vi "Check Filter Repositioning Status.vi"(0 "Session Handle in":T1, 11 "error in (no error)":errorcluster) -> (4 "Session Handle out":T1, 6 "Success?":bool, 15 "error out":errorcluster)   [LabVIEW 2015, in "PAS.lvclass"]
uses:
  PAS.lvclass
  Typedefs/Session Handle.ctl
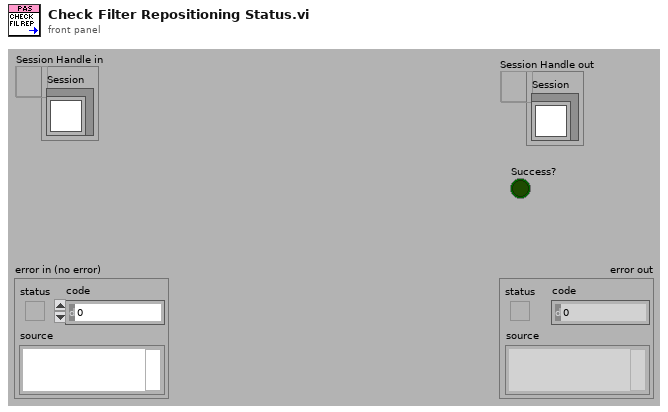
[diagram p1: front panel]
types:
  T1 = typedef "PAS.lvclass/Session Handle.ctl" = refnum<data-value>
  T2 = typedef "XNET Frame CAN.ctl" = cluster{"timestamp":timestamp, "payload":u8[], "identifier":u32, "type":T3, "extended?":bool, "echo?":bool}
  T3 = typedef "XNET Frame Type CAN.ctl" = u8
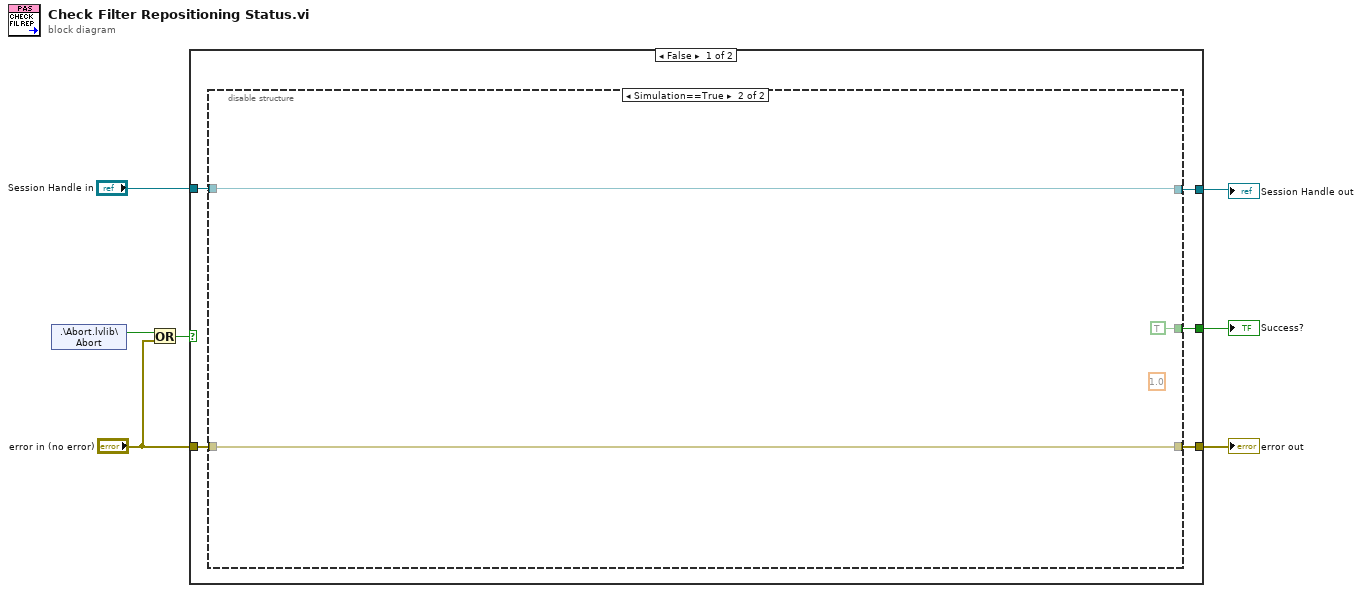
[diagram p0: block diagram]
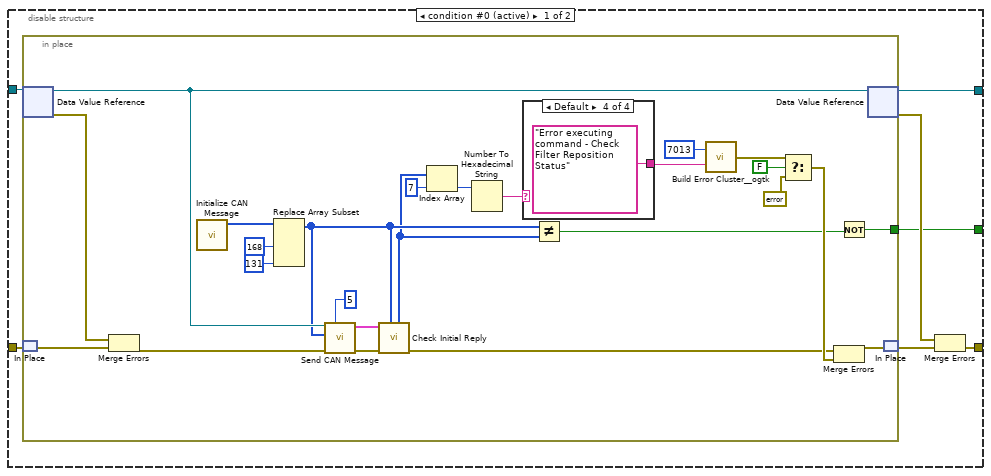
[diagram p2: hidden frame]
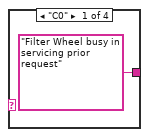
[diagram p3: hidden frame]
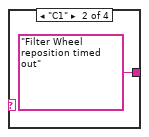
[diagram p4: hidden frame]
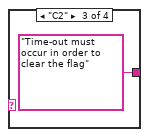
[diagram p5: hidden frame]
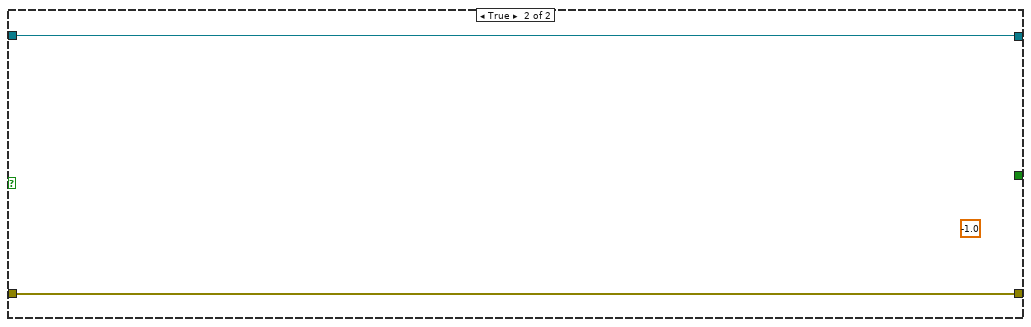
[diagram p6: hidden frame]
diagram:
  n1 = shared-variable ".\\Abort.lvlib\\Abort"() -> (w4:bool)  [unwired: 1 in, 1 out]
  n2 = Or(x=w4, y="error in (no error)") -> (x .or. y?=w2:bool)
  n3 = case shown="False" w2 {
    tunnel: [w12 w53] -> w6
    tunnel: [w11 w52] -> w5
    tunnel: "Session Handle in" -> [w10 w53]
    tunnel: "error in (no error)" -> [w9 w52]
    tunnel: [w8 _] -> w1
    frame False {
      n4 = disable-structure shown="Simulation==True" {
        disable-tunnel: [w19 w51] -> w12
        disable-tunnel: [w16 w50] -> w11
        disable-tunnel: w10 -> [w15 w51]
        disable-tunnel: w9 -> [w14 w50]
        disable-tunnel: [w13 TRUE] -> w8
        frame condition #0 (active) {
          n5 = in-place {
            in-place-border: [w34] -> w13
            n6 = in-place-dvr #1(w15) -> (w37:refnum<class "PAS.lvclass">, w41:errorcluster)
            n7 = in-place-match #2(w14) -> (w40:errorcluster)
            n8 = Merge Errors(w41, w40) -> (w36:errorcluster)
            n9 = call "Initialize CAN Message.vi"() -> ("Initial Payload"=w42:u8[])  [unwired: 11 in]
            n10 = Replace Array Subset(array=w42, new element #1=u8 168 ("new element/subarray"), new element #2=u8 131 ("new element/subarray")) -> (w29:u8[])  [unwired: 2 in]
            n11 = call "Send CAN Message.vi"("Number of Retries"=5, "error in (no error)"=w36, "payload"=w29, "Gas In"=w37) -> ("error out"=w21:errorcluster, "Reply"=w38:T2[])  [unwired: 5 in, 1 out]
            n12 = call "Check Initial Reply.vi"("Write Message"=w29, "error in (no error)"=w21, "Reply"=w38) -> ("error out"=w20:errorcluster, "Whole Payload"=w27:u8[])  [unwired: 5 in, 2 out]
            n13 = Index Array(array=w27, index=7) -> (element=w25:u8)
            n14 = Number To Hexadecimal String(2:w25) -> (0:w23:string)  [unwired: 1 in]
            n15 = case shown="Default" w23 {
              tunnel: ["Filter Wheel busy in servicing prior request" "Filter Wheel reposition timed out" "Time-out must occur in order to clear the flag" "Error executing command - Check Filter Reposition Status"] -> w22
              frame "C0" {
              }
              frame "C1" {
              }
              frame "C2" {
              }
              frame Default {
              }
            }
            n16 = Not Equal?(x=w29, y=w27) -> (x != y?=w28:bool)
            n17 = call <userlib>:"Build Error Cluster__ogtk.vi"("String to Prepend to source (\"\")"=w22, "code"=7013) -> ("error out"=w33:errorcluster)
            n18 = Select(t=w33, s=FALSE, f=errorcluster {"status"=FALSE, "code"=0, "source"=""}) -> (s? t:f=w30:errorcluster)
            n19 = Merge Errors(w20, w30) -> (w43:errorcluster)
            n20 = Not(x=w28) -> (.not. x?=w34:bool)
            n21 = in-place-dvr #1(w37) -> (w19:T1, w17:errorcluster)
            n22 = in-place-match #2(w43) -> (w18:errorcluster)
          }
          n23 = Merge Errors(w17, w18) -> (w16:errorcluster)
        }
        frame condition #1 {
          (unwired) 1.0
        }
      }
    }
    frame True {
      (unwired) -1.0
    }
  }
  "Session Handle out" <- w6
  "error out" <- w5
  "Success?" <- w1
